vi "Serial data.vi"(8 "error in":errorcluster, 10 "Serial Number":string, 11 "refnum in":refnum<file>) -> (0 "error out":errorcluster, 3 "refnum out":refnum<file>)   [LabVIEW 2018]
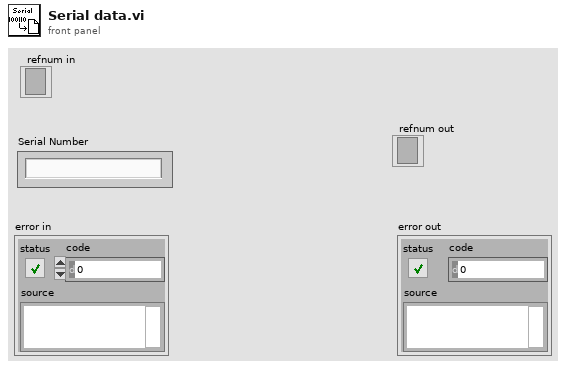
[diagram p1: front panel]
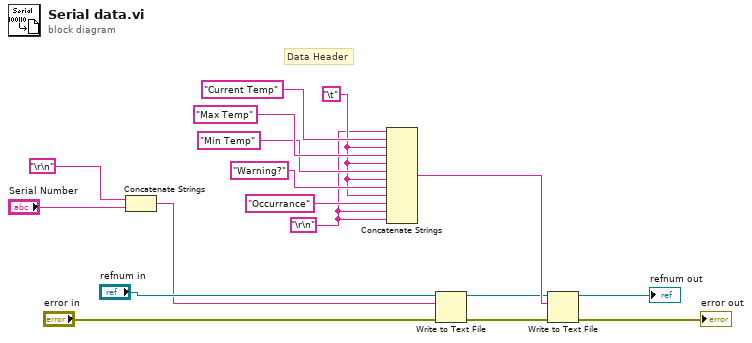
[diagram p0: block diagram]
diagram:
  w4 = "\r\n"
  w13 = "\t"
  # "Data Header"
  n1 = Concatenate Strings("\r\n", "Serial Number") -> (w3:string)
  n2 = Concatenate Strings(w4, "Current Temp" ("string"), w13, "Max Temp" ("string"), w13, "Min Temp" ("string"), w13, "Warning?" ("string"), w13, "Occurrance" ("string"), w4, w4) -> (w10:string)
  n3 = Write to Text File(file (use dialog)="refnum in", text=w3, error in="error in") -> (refnum out=w9:refnum<file>, error out=w8:errorcluster)  [unwired: 1 in, 1 out]
  n4 = Write to Text File(file (use dialog)=w9, text=w10, error in=w8) -> (refnum out=→"refnum out":refnum<file>, error out=→"error out":errorcluster)  [unwired: 1 in, 1 out]
